vi "UpCaculateCellROI.vi"() -> (1 "total":dbl[][](array[numeric]), 2 "CellROI":cluster{dbl, dbl, dbl, dbl}[][](array[cluster]), 3 "Score":dbl[](array[numeric]))   [LabVIEW 2019]
uses:
  Ctrl/UpEnum_VisionCalibSet_Act.ctl
panel:
  in  "y":dbl=130.0 format="%#_13g"
  out "subarray 3":dbl[](array[numeric])
  out "subarray 2":dbl[](array[numeric])
  out "subarray":dbl[](array[numeric])
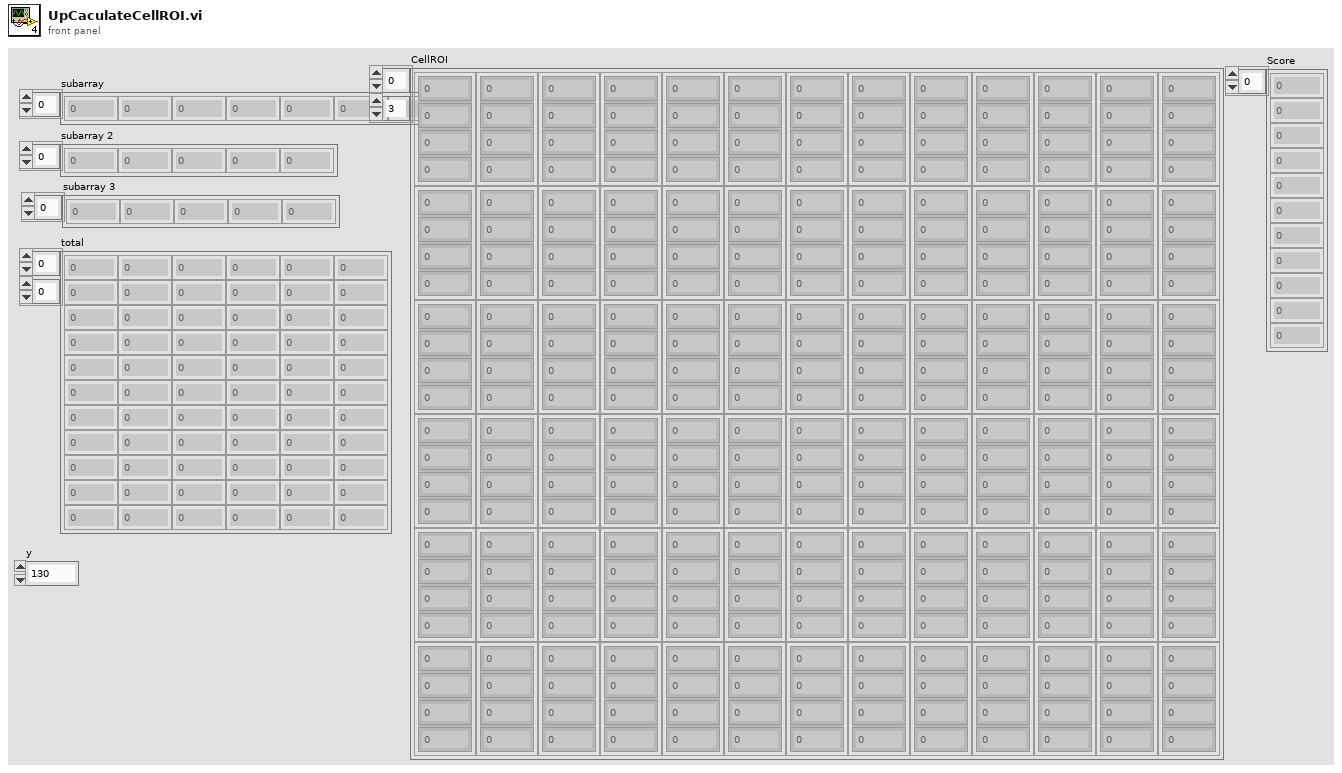
[diagram p1: front panel]
types:
  T1 = cluster{"XY_ATray":cluster{"X":i32, "Y":i32}, "Initial color":u32, "FinalColor":u32}
  T2 = typedef "IMAQ Rectangle" = cluster{"Left":i32, "Top":i32, "Right":i32, "Bottom":i32, "Rotation":dbl}
  T3 = typedef "UpEnum_VisionCalibSet_Act.ctl" = enum16{"initial", "initialref", "save", "load", "UpDataToUI", "write", "read"}
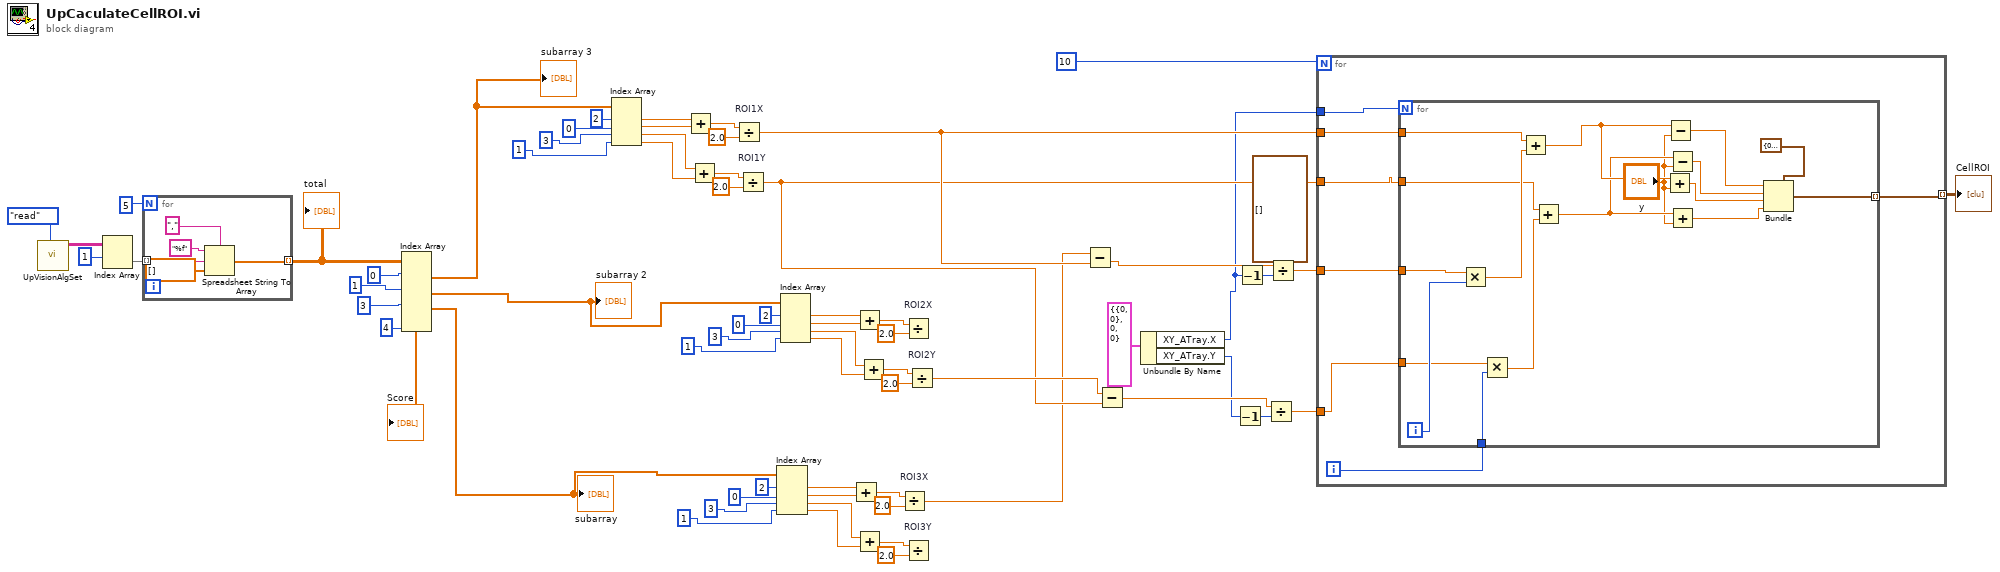
[diagram p0: block diagram]
diagram:
  (unwired) T2[] []
  n1 = call "UpVisionAlgSet.vi"("Enum"=UpEnum_VisionCalibSet_Act."read") -> ("Table Control"=w63:string[][])  [unwired: 8 in, 2 out]
  n2 = Index Array(array=w63, index (row)=1) -> (element=w62:string[])  [unwired: 1 in]
  n3 = for {
    N: 5 -> [_]
    tunnel: w62 -> [w69] mode=indexing
    tunnel: [w67] -> w60 mode=indexing
    n4 = Spreadsheet String To Array(delimiter (Tab)=",", format string="%f", spreadsheet string=w69, array type (2D Dbl)=dbl[] []) -> (array=w67:dbl[])
  }
  "total" <- w60
  n5 = Index Array(array=w60, index (row) #1=0 ("disabled index (col)"), index (row) #2=1 ("index (col)"), index (row) #3=3 ("index (col)"), index (col) #4=4 ("disabled index (col)")) -> (element #1=w56:dbl[], element #2=w31:dbl[], element #3=w18:dbl[], element #4=→"Score":dbl[])  [unwired: 4 in]
  "subarray" <- w18
  "subarray 2" <- w31
  "subarray 3" <- w56
  n6 = Index Array(array=w56, index #1=2 ("index"), index #2=0 ("index"), index #3=3 ("index"), index #4=1 ("index")) -> (element #1=w50:dbl, element #2=w51:dbl, element #3=w45:dbl, element #4=w44:dbl)
  n7 = Add(x=w50, y=w51) -> (x+y=w49:dbl)
  n8 = Add(x=w45, y=w44) -> (x+y=w46:dbl)
  n9 = Divide "ROI1X"(x=w49, y=2.0) -> (x/y=w11:dbl)
  n10 = Divide "ROI1Y"(x=w46, y=2.0) -> (x/y=w10:dbl)
  n11 = Index Array(array=w18, index #1=2 ("index"), index #2=0 ("index"), index #3=3 ("index"), index #4=1 ("index")) -> (element #1=w25:dbl, element #2=w26:dbl, element #3=w20:dbl, element #4=w19:dbl)
  n12 = Index Array(array=w31, index #1=2 ("index"), index #2=0 ("index"), index #3=3 ("index"), index #4=1 ("index")) -> (element #1=w37:dbl, element #2=w36:dbl, element #3=w42:dbl, element #4=w43:dbl)
  n13 = Add(x=w25, y=w26) -> (x+y=w24:dbl)
  n14 = Add(x=w37, y=w36) -> (x+y=w38:dbl)
  n15 = Add(x=w20, y=w19) -> (x+y=w21:dbl)
  n16 = Add(x=w42, y=w43) -> (x+y=w41:dbl)
  n17 = Divide "ROI3X"(x=w24, y=2.0) -> (x/y=w6:dbl)
  n18 = Divide "ROI2X"(x=w38, y=2.0) -> ()  [unwired: 1 out]
  n19 = Divide "ROI3Y"(x=w21, y=2.0) -> ()  [unwired: 1 out]
  n20 = Divide "ROI2Y"(x=w41, y=2.0) -> (x/y=w17:dbl)
  n21 = Subtract(x=w6, y=w11) -> (x-y=w16:dbl)
  n22 = Subtract(x=w17, y=w10) -> (x-y=w13:dbl)
  n23 = Unbundle By Name(T1 {"XY_ATray"={"X"=0, "Y"=0}, "Initial color"=0, "FinalColor"=0} ("input cluster")) -> ("XY_ATray.X"=w8:i32, "XY_ATray.Y"=w7:i32)
  n24 = Decrement(x=w7) -> (x-1=w14:i32)
  n25 = Decrement(x=w8) -> (x-1=w15:i32)
  n26 = Divide(x=w13, y=w14) -> (x/y=w12:dbl)
  n27 = Divide(x=w16, y=w15) -> (x/y=w9:dbl)
  n28 = for {
    N: 10 -> [_]
    tunnel: w12 -> [w73]
    tunnel: w11 -> [w77]
    tunnel: w10 -> [w76]
    tunnel: w9 -> [w75]
    tunnel: w8 -> [w72]
    tunnel: [w71] -> w4 mode=indexing
    i -> [w74]
    n29 = for {
      N: w72 -> [_]
      tunnel: w77 -> [w94]
      tunnel: w76 -> [w90]
      tunnel: w75 -> [w93]
      tunnel: w74 -> [w89]
      tunnel: w73 -> [w87]
      tunnel: [w78] -> w71 mode=indexing
      i -> [w92]
      n30 = Multiply(x=w93, y=w92) -> (x*y=w91:dbl)
      n31 = Multiply(x=w87, y=w89) -> (x*y=w88:dbl)
      n32 = Add(x=w94, y=w91) -> (x+y=w86:dbl)
      n33 = Add(x=w90, y=w88) -> (x+y=w85:dbl)
      n34 = Add(x=w86, y="y") -> (x+y=w81:dbl)
      n35 = Subtract(x=w86, y="y") -> (x-y=w83:dbl)
      n36 = Subtract(x=w85, y="y") -> (x-y=w82:dbl)
      n37 = Add(x=w85, y="y") -> (x+y=w80:dbl)
      n38 = Bundle(cluster=cluster{dbl, dbl, dbl, dbl} {0.0, 0.0, 0.0, 0.0} ("output cluster"), w83, w82, w81, w80) -> (w78:cluster{dbl, dbl, dbl, dbl})
    }
  }
  "CellROI" <- w4
